vi "Standardize Angle in Degrees.vi"(3 "angle in (deg)":dbl, 4 "range (-180 to 180)":T1=enum."-180 to 180") -> (5 "angle out (deg)":dbl)   [LabVIEW 2017, in "NI_Robotics Utilities.lvlib"]
doc: "Wraps an angle in degrees to be within a specific range.\n\nThis VI is deprecated. Use <vi.lib>\\Analysis\\coordinate.llb\\Wrap Angle.vi instead."
uses:
  <vilib>/robotics/Utilities/NI_Robotics Utilities.lvlib
  <vilib>/robotics/Utilities/Angle Range_Degrees.ctl
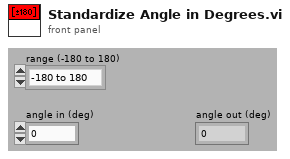
[diagram p1: front panel]
types:
  T1 = typedef "NI_Robotics Utilities.lvlib/Angle Range_Degrees.ctl" = enum16{"none", "-180 to 180", "0 to 360"}
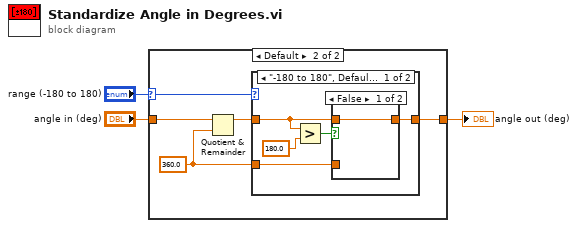
[diagram p0: block diagram]
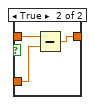
[diagram p3: hidden frame]
diagram:
  n1 = case shown="Default" "range (-180 to 180)" {
    selector: "range (-180 to 180)" -> [_ w5]
    tunnel: "angle in (deg)" -> [w4 w8]
    tunnel: [w4 w7] -> w2
    frame "none" {
    }
    frame Default {
      w6 = 360.0
      n2 = Quotient & Remainder(x=w8, y=w6) -> (x-y*floor(x/y)=w9:dbl)  [unwired: 1 out]
      n3 = case shown="\"-180 to 180\", Default" w5 {
        tunnel: w9 -> [w14 w19]
        tunnel: [w12 w19] -> w7
        tunnel: w6 -> [w10 _]
        frame "-180 to 180", Default {
          n4 = Greater?(x=w14, y=180.0) -> (0:w13:bool)
          n5 = case shown="False" w13 {
            tunnel: w14 -> [w15 w18]
            tunnel: [w15 w17] -> w12
            tunnel: w10 -> [_ w16]
            frame False {
            }
            frame True {
              n6 = Subtract(x=w18, y=w16) -> (x-y=w17:dbl)
            }
          }
        }
        frame "0 to 360" {
        }
      }
    }
  }
  "angle out (deg)" <- w2
